vi "UploadArduino.vi"(10 "serial port":string, 11 "Sketch.ino":string="WifiBackpack.ino") -> (2 "standard error":string, 3 "standard output":string)   [LabVIEW 2020]
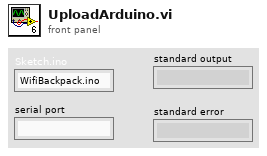
[diagram p1: front panel]
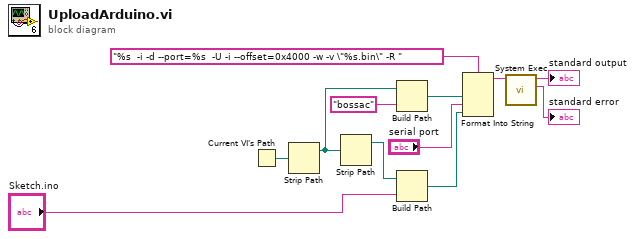
[diagram p0: block diagram]
diagram:
  n1 = Current VI's Path() -> (path=w2:path)
  n2 = Strip Path(path=w2) -> (stripped path=w1:path)  [unwired: 1 out]
  n3 = Strip Path(path=w1) -> (stripped path=w3:path)  [unwired: 1 out]
  n4 = Build Path(base path=w1, name or relative path="bossac" ("Sketch.ino")) -> (appended path=w4:path)
  n5 = Build Path(base path=w3, name or relative path="Sketch.ino") -> (appended path=w8:path)
  n6 = Format Into String(format string="%s  -i -d --port=%s  -U -i --offset=0x4000 -w -v \"%s.bin\" -R ", w4, "serial port", w8) -> (resulting string=w6:string)  [unwired: 2 in, 1 out]
  n7 = call <vilib>:"System Exec.vi"("command line"=w6) -> ("standard error"=→"standard error":string, "standard output"=→"standard output":string)  [unwired: 7 in, 2 out]
